vi "Compass on new GIC parallel.vi"(11 "GIC Input 2":T1={"     Use ?\nOff       On"=[FALSE, TRUE, FALSE, TRUE], "Mode:"=FALSE, "Extra Port"="", "Hokuyo Port"="COM7", "Tx Prop  Port"="COM6", "Compass Port"="", "GPS Port"="", "Num of WPs"=0, "WP Lats and Longs"={"WP Lats"=[], "WP Longs"=[]}, "Obst Lats and Longs"={"Obst Lats"=[], "Obst Longs"=[]}, "Parameters"=[], "GPS Data"=[], "Compass"=0.0, "LMS Vector"=[], "Vision Vector"=[], "Direction Cmd"=0.0, "Speed Cmd"=0.0, "WP Vector"=[], "WP Number"=0, "Extra"=0, "SW Map"=[], "Path Cluster"={"Path x node"=[], "Path y node"=[]}, "Sim Course"=[]} {"Obst Lats and Longs"."Obst Longs" format="%#_8g"; "Obst Lats and Longs"."Obst Lats" format="%#_8g"}) -> (3 "GIC Output 2":T1={"     Use ?\nOff       On"=[FALSE, TRUE, FALSE, TRUE], "Mode:"=FALSE, "Extra Port"="", "Hokuyo Port"="COM7", "Tx Prop  Port"="COM6", "Compass Port"="", "GPS Port"="", "Num of WPs"=0, "WP Lats and Longs"={"WP Lats"=[], "WP Longs"=[]}, "Obst Lats and Longs"={"Obst Lats"=[], "Obst Longs"=[]}, "Parameters"=[], "GPS Data"=[], "Compass"=0.0, "LMS Vector"=[], "Vision Vector"=[], "Direction Cmd"=0.0, "Speed Cmd"=0.0, "WP Vector"=[], "WP Number"=0, "Extra"=0, "SW Map"=[], "Path Cluster"={"Path x node"=[], "Path y node"=[]}, "Sim Course"=[]} {"Obst Lats and Longs"."Obst Longs" format="%#_8g"; "Obst Lats and Longs"."Obst Lats" format="%#_8g"})   [LabVIEW 2014]
uses:
  Global_vars.vi
panel:
  out "compass in":dbl
  out "compass out":dbl
  # "Compass on new GIC parallel"
  # "Compass on New GIC A"
  # "Input:"
  # "Output:"
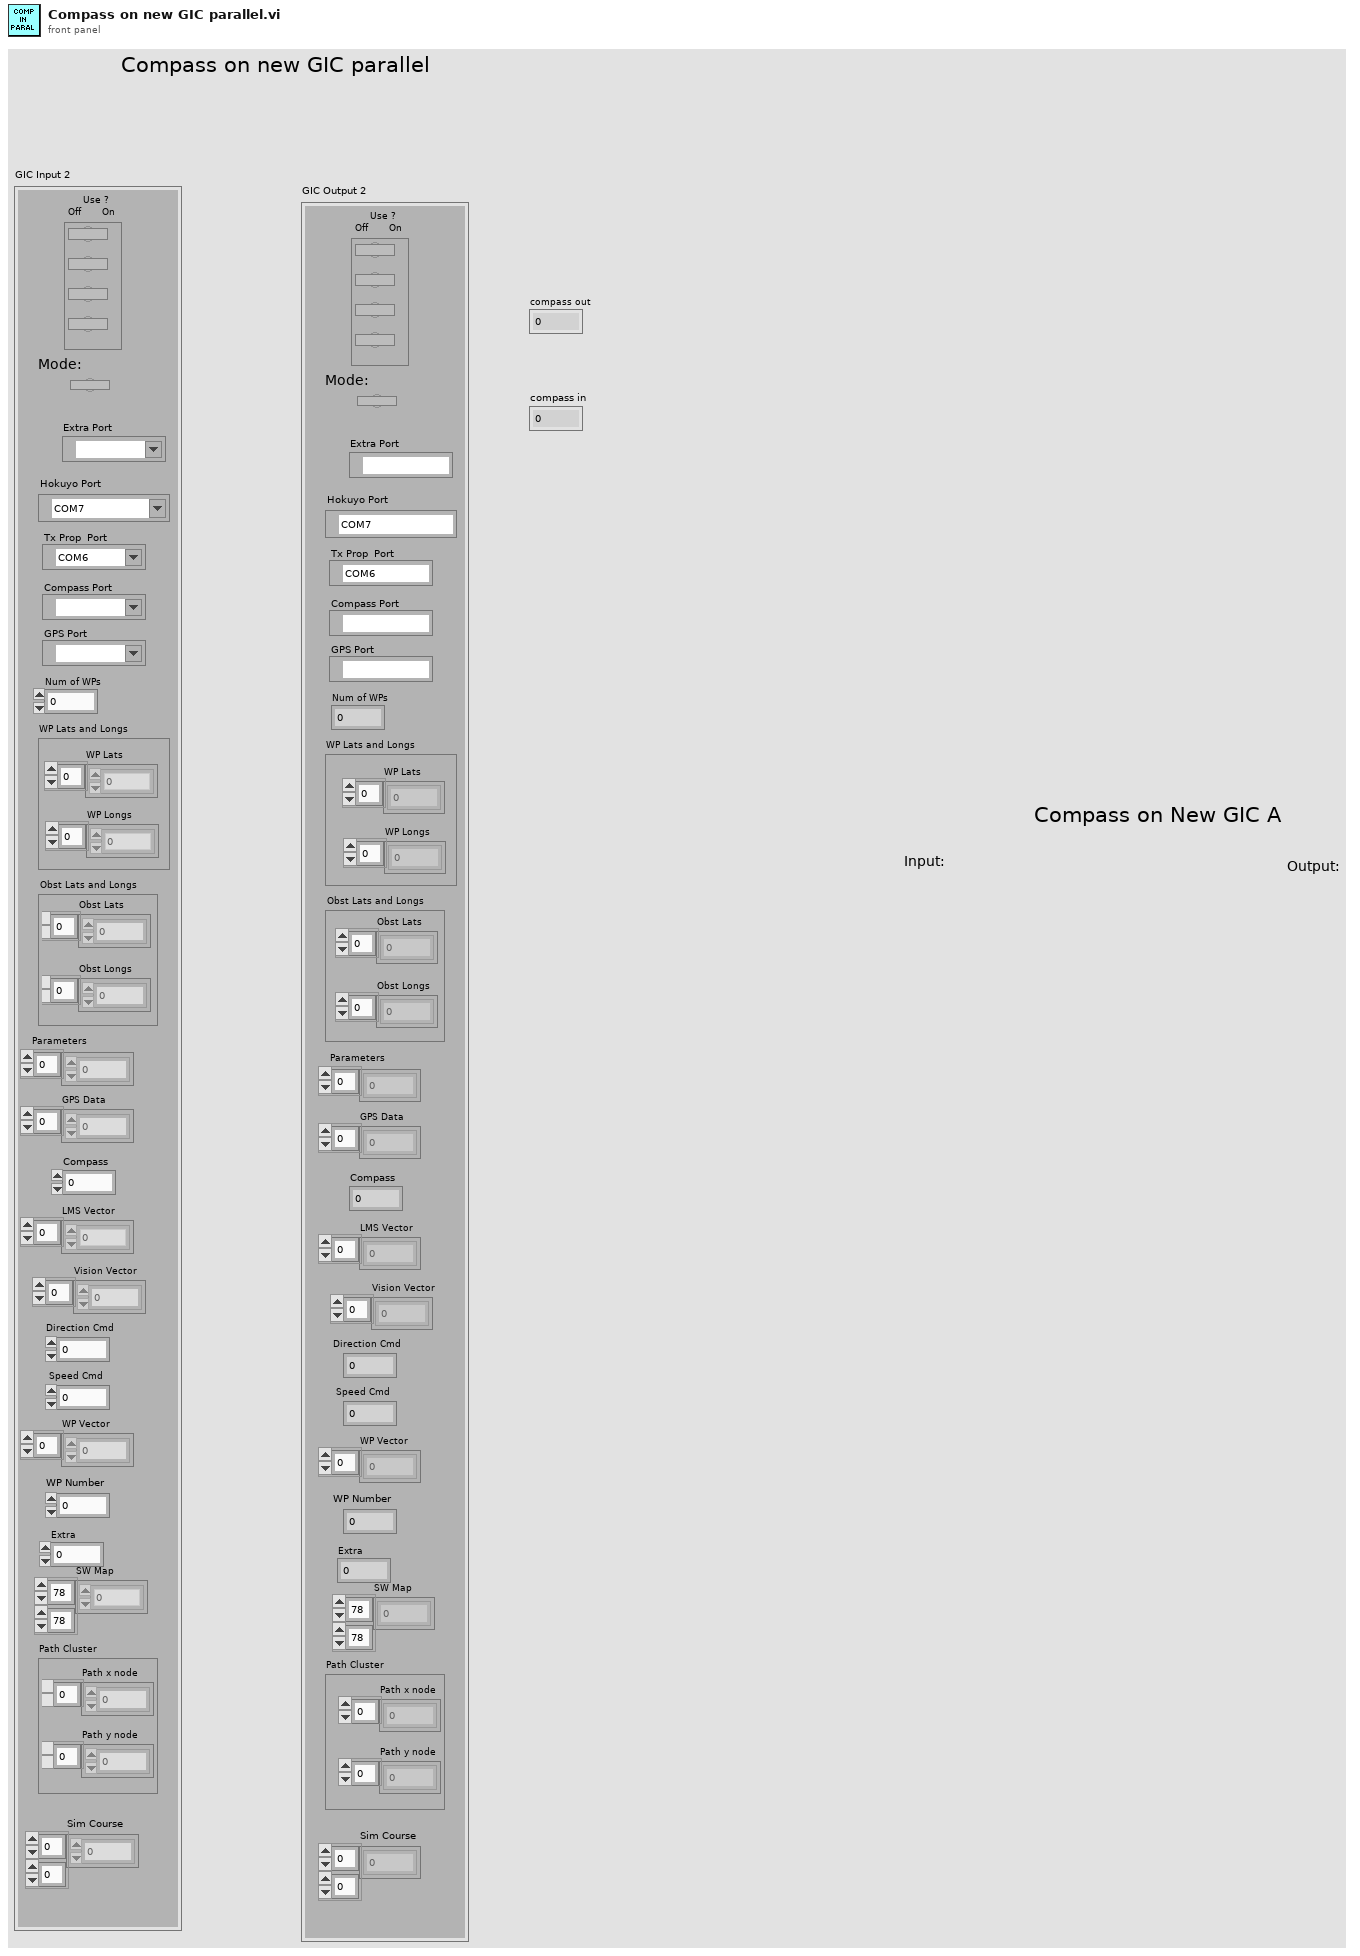
[diagram p1: front panel]
types:
  T1 = cluster{"     Use ?\nOff       On":bool[], "Mode:":bool, "Extra Port":refnum<visa-resource-name>, "Hokuyo Port":refnum<visa-resource-name>, "Tx Prop  Port":refnum<visa-resource-name>, "Compass Port":refnum<visa-resource-name>, "GPS Port":refnum<visa-resource-name>, "Num of WPs":i16, "WP Lats and Longs":cluster{"WP Lats":dbl[], "WP Longs":dbl[]}, "Obst Lats and Longs":cluster{"Obst Lats":dbl[], "Obst Longs":dbl[]}, "Parameters":dbl[], "GPS Data":dbl[], "Compass":dbl, "LMS Vector":dbl[], "Vision Vector":dbl[], "Direction Cmd":dbl, "Speed Cmd":dbl, "WP Vector":dbl[], "WP Number":i32, "Extra":i16, "SW Map":i32[][], "Path Cluster":cluster{"Path x node":dbl[], "Path y node":dbl[]}, "Sim Course":i8[][]}
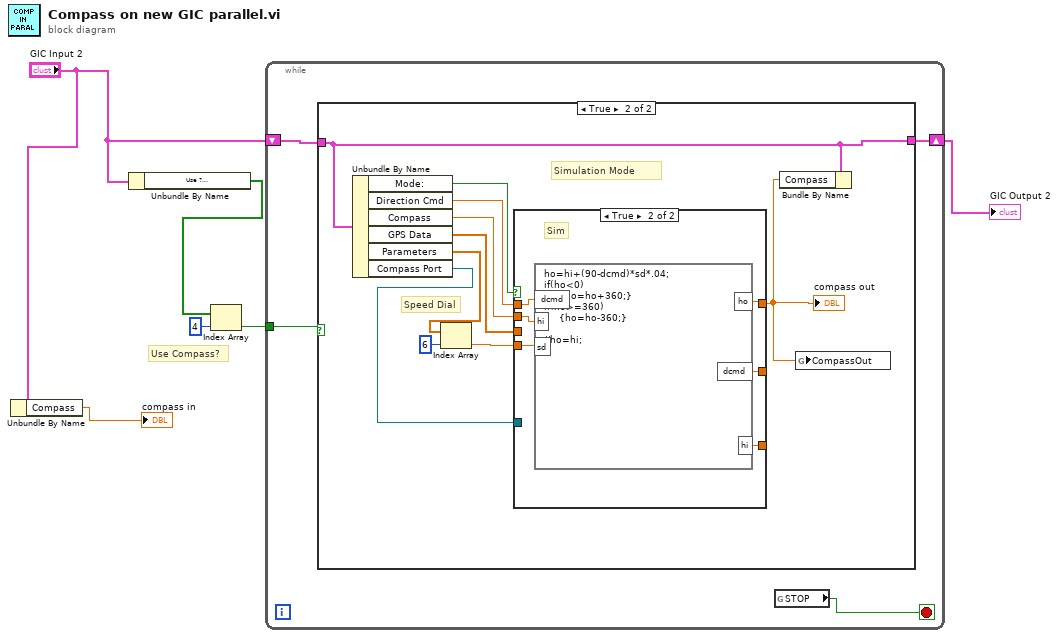
[diagram p0: block diagram]
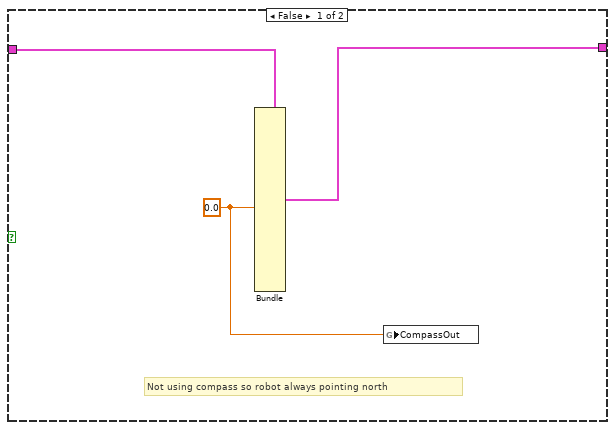
[diagram p2: hidden frame]
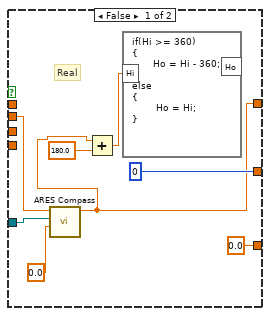
[diagram p3: hidden frame]
diagram:
  # "Use Compass?"
  n1 = Unbundle By Name("GIC Input 2") -> ("Compass"=→"compass in":dbl)
  n2 = Unbundle By Name("GIC Input 2") -> ("Use ?\nOff       On"=w6:bool[])
  n3 = Index Array(array=w6, index=4) -> (element=w4:bool)
  n4 = while {
    tunnel: w4 -> [w8]
    shift-right: [w9] -> w3
    shift-left: "GIC Input 2" -> [w10]
    stop <- w7 stop-if-true
    n5 = case shown="True" w8 {
      tunnel: w10 -> [w13 w17]
      tunnel: [w12 w17] -> w9
      frame False {
        w11 = 0.0 ("Compass")
        # "Not using compass so robot always pointing north"
        n6 = Bundle(cluster=w13, "Compass"=w11) -> (w12:T1)  [unwired: 22 in]
        n7 = global write "Global_vars.vi" "CompassOut"(w11) -> ()
      }
      frame True {
        # "Simulation Mode"
        # "Speed Dial"
        n8 = Unbundle By Name(w17) -> ("Mode:"=w22:bool, "Direction Cmd"=w14:dbl, "Compass"=w15:dbl, "GPS Data"=w23:dbl[], "Parameters"=w21:dbl[], "Compass Port"=w18:refnum<visa-resource-name>)
        n9 = Index Array(array=w21, index=6) -> (element=w19:dbl)
        n10 = case shown="True" w22 {
          tunnel: w14 -> [_ w36]
          tunnel: w15 -> [w29 w35]
          tunnel: [w24 w37] -> w16
          tunnel: w23 -> [_ _]
          tunnel: w19 -> [_ w34]
          tunnel: [0 w33] -> _
          tunnel: [0.0 ("hi") w32] -> _
          tunnel: w18 -> [w28 _]
          frame False {
            # "Real"
            n11 = call "ARES Compass.vi"("Input time of last compass read"=0.0, "Compass Com Port"=w28, "Compass In"=w29) -> ("Compass Out"=w24:dbl)  [unwired: 6 in, 1 out]
            n12 = Add(x=w24, y=180.0) -> (x+y=w25:dbl)
            n13 = formula code="if(Hi >= 360)\n{\n       Ho = Hi - 360;\n}\nelse\n{\n        Ho = Hi;\n}"("Hi"=w25) -> ()  [unwired: 1 out]
          }
          frame True {
            # "Sim"
            n14 = formula code="ho=hi+(90-dcmd)*sd*.04;\nif(ho<0)\n     {ho=ho+360;}\nif(ho>=360)\n     {ho=ho-360;}\n\n//ho=hi;"("dcmd"=w36, "hi"=w35, "sd"=w34) -> ("ho"=w37:dbl, "dcmd"=w33:dbl, "hi"=w32:dbl)
          }
        }
        "compass out" <- w16
        n15 = Bundle By Name(cluster=w17, "Compass"=w16) -> ()  [unwired: 1 out]
        n16 = global write "Global_vars.vi" "CompassOut"(w16) -> ()
      }
    }
    n17 = global read "Global_vars.vi" "STOP"() -> (w7:bool)
  }
  "GIC Output 2" <- w3
